vi "TimedLoop.vi"() -> ()   [LabVIEW 2017]
panel:
  out "Max":i32
  out "Time":i32
  out "Z Position":i32
  out "X Position":i32
  out "Y Position":i32
  out "Speed Z":i32
  out "Speed X":i32
  out "Speed Y":i32
  out "Numeric 3":i32
  out "Numeric 2":i32
  out "Numeric":i32
  in  "Array 3":dbl[](array[numeric])
  in  "Array 2":dbl[](array[numeric])
  in  "Array":dbl[](array[numeric])
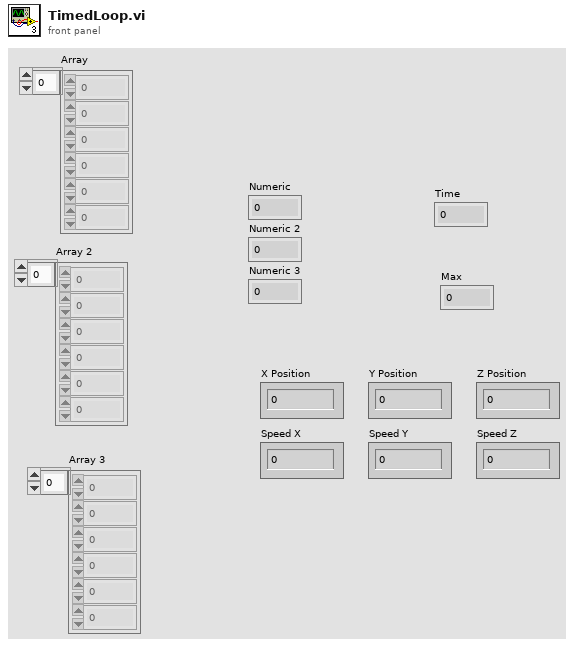
[diagram p1: front panel]
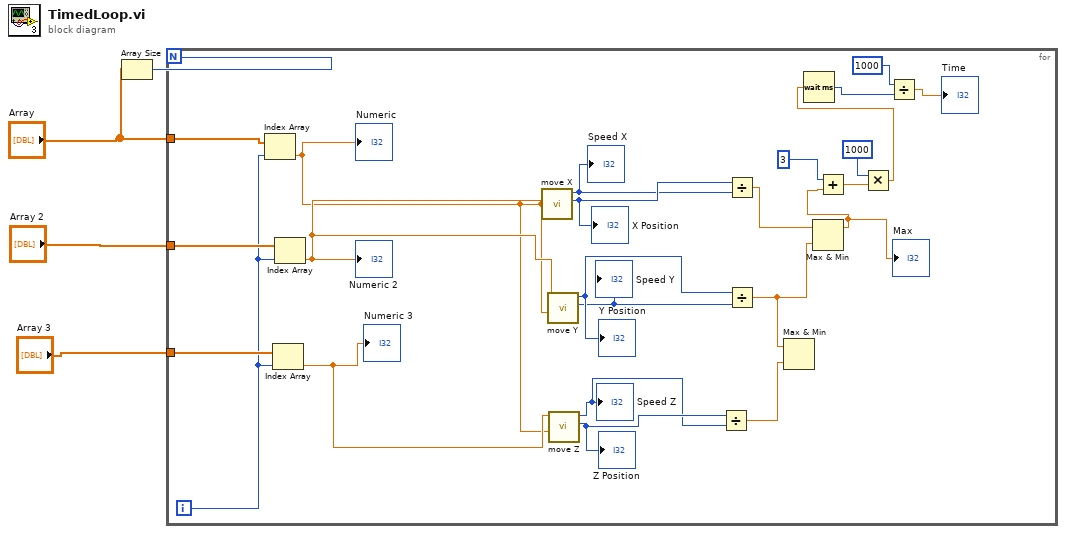
[diagram p0: block diagram]
diagram:
  n1 = Array Size(array="Array") -> (size(s)=w4:i32)
  n2 = for {
    N: w4 -> [_]
    tunnel: "Array" -> [w28]
    tunnel: "Array 2" -> [w27]
    tunnel: "Array 3" -> [w26]
    i -> [w25]
    n3 = Index Array(array=w28, index=w25) -> (element=w22:dbl)
    "Numeric" <- w22
    n4 = Index Array(array=w26, index=w25) -> (element=w23:dbl)
    "Numeric 3" <- w23
    n5 = Index Array(array=w27, index=w25) -> (element=w24:dbl)
    "Numeric 2" <- w24
    n6 = call "move X.vi"("y mm"=w24, "x mm"=w22) -> ("X Position"=w21:i32, "Speed X"=w20:i32)  [unwired: 8 in]
    "Speed X" <- w20
    "X Position" <- w21
    n7 = call "move Y.vi"("x mm"=w22, "y mm"=w24) -> ("Y Speed"=w18:i32, "Y Position"=w19:i32)  [unwired: 8 in]
    "Speed Y" <- w18
    "Y Position" <- w19
    n8 = call "move Z.vi"("x mm"=w22, "z mm"=w23) -> ("Z Position"=w17:i32, "Z Speed"=w16:i32)  [unwired: 8 in]
    "Speed Z" <- w16
    "Z Position" <- w17
    n9 = Divide(x=w17, y=w16) -> (x/y=w15:dbl)
    n10 = Divide(x=w21, y=w20) -> (x/y=w14:dbl)
    n11 = Divide(x=w19, y=w18) -> (x/y=w13:dbl)
    n12 = Max & Min(x=w13, y=w15) -> ()  [unwired: 2 out]
    n13 = Max & Min(x=w14, y=w13) -> (max(x,y)=w11:dbl)  [unwired: 1 out]
    "Max" <- w11
    n14 = Add(x=3, y=w11) -> (x+y=w10:dbl)
    n15 = Multiply(x=1000, y=w10) -> (x*y=w8:dbl)
    n16 = Wait (ms)(milliseconds to wait=w8) -> (millisecond timer value=w6:u32)
    n17 = Divide(x=1000, y=w6) -> (x/y=→"Time":dbl)
  }
